vi "Math Rolling Buffer (by ref).vi"(0 "New Data In":sgl[][](array[numeric]), 1 "# Pts Read":u32, 3 "Number of Channels":i32=1, 4 "Sample Rate":dbl=2000.0, 5 "error in (no error)":errorcluster, 7 "Config.Test Limits":T1[](array[typedef]), 9 "Coefficients":cluster{"Coefficients":dbl[]}[](array[cluster]), 10 "Mode (Read)":T2=enum."Read") -> (14 "Buffer Out":sgl[][](array[numeric]), 15 "Data Indexes":i32[](array[numeric]), 16 "RMS":sgl[][](array[numeric]), 17 "PK-PK":sgl[][](array[numeric]), 18 "Frequency Data":sgl[][](array[numeric]), 19 "error out":errorcluster)   [LabVIEW 2019]
uses:
  Type Defs and Controls/Functional Global Control.ctl
  Type Defs and Controls/Test Limits.ctl
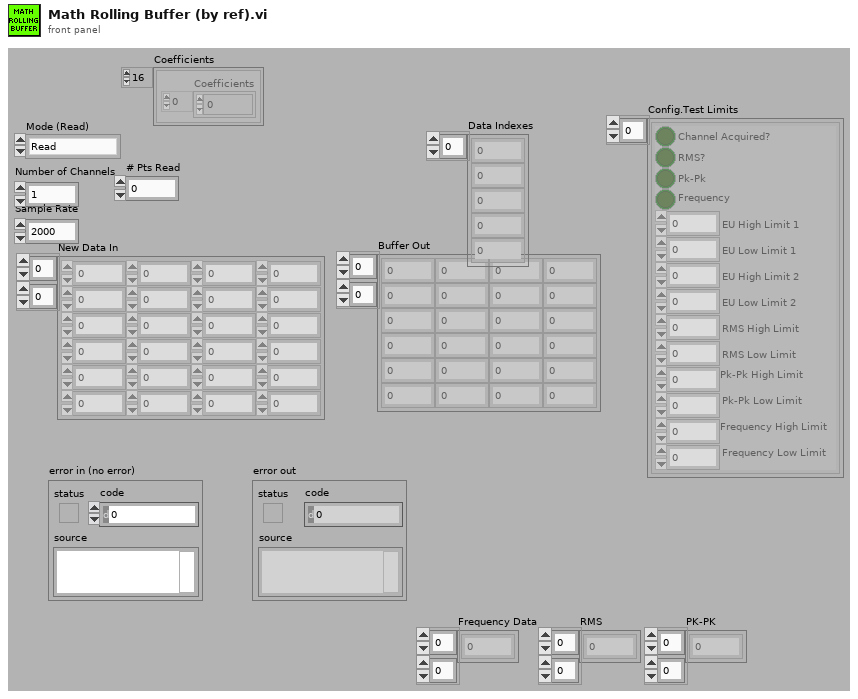
[diagram p1: front panel]
types:
  T1 = typedef "Test Limits.ctl" = cluster{"Channel Acquired?":bool, "RMS?":bool, "Pk-Pk":bool, "Frequency":bool, "EU High Limit 1":dbl, "EU Low Limit 1":dbl, "EU High Limit 2":dbl, "EU Low Limit 2":dbl, "RMS High Limit":dbl, "RMS Low Limit":dbl, "Pk-Pk High Limit ":dbl, "Pk-Pk Low Limit":dbl, "Frequency High Limit":dbl, "Frequency Low Limit":dbl}
  T2 = typedef "Functional Global Control.ctl" = enum16{"Nothing", "Init", "Read", "Write"}
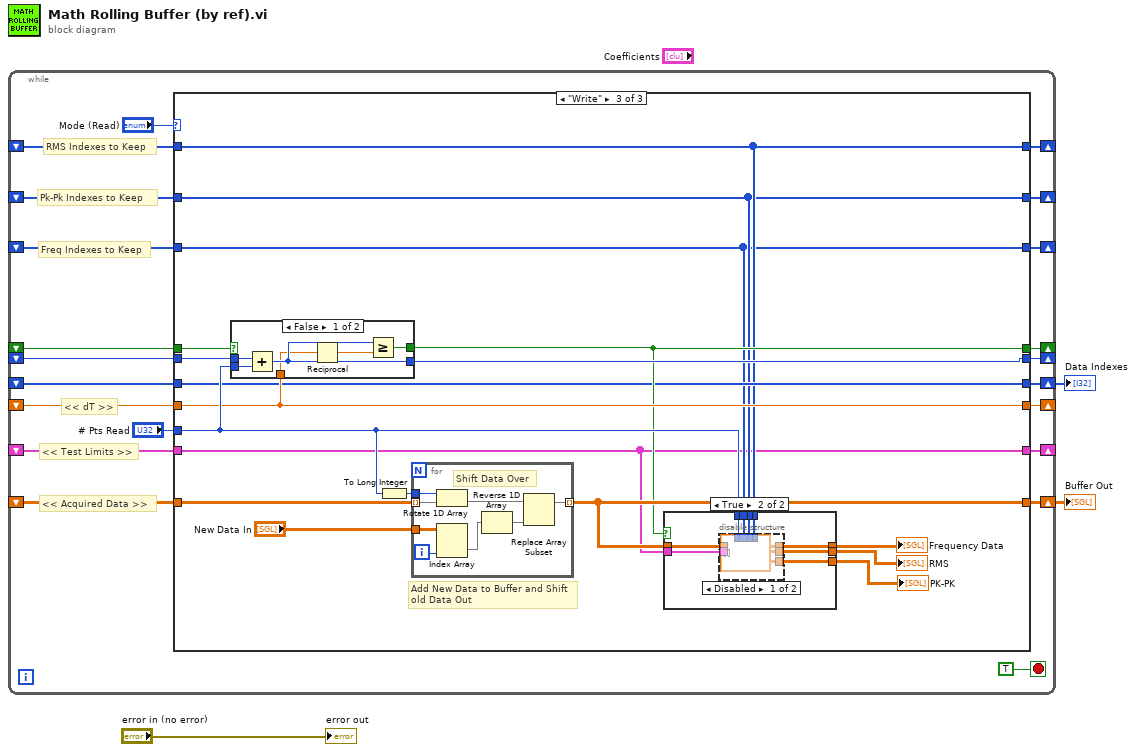
[diagram p0: block diagram]
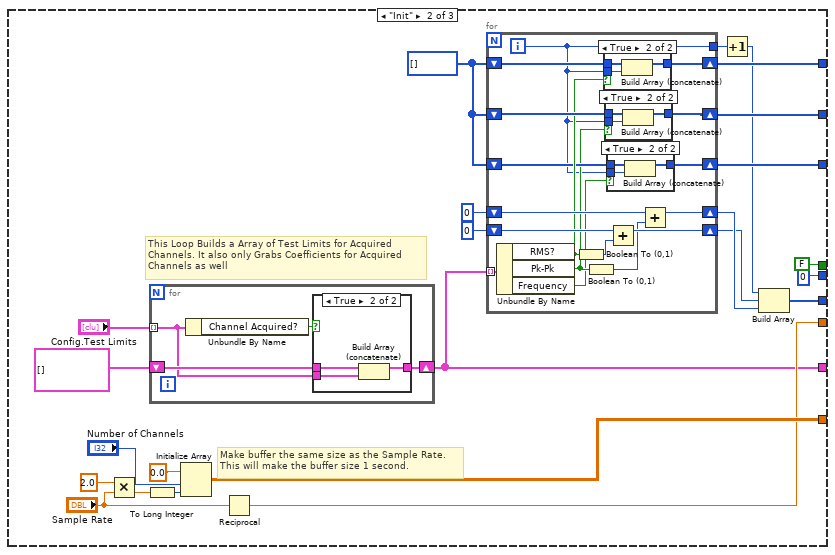
[diagram p3: hidden frame]
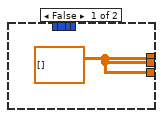
[diagram p8: hidden frame]
diagram:
  n1 = while {
    shift-right: [w22] -> w3
    shift-left: _ -> [w21]
    shift-right: [w20] -> _
    shift-left: _ -> [w19]
    shift-right: [w17] -> _
    shift-left: _ -> [w18]
    shift-right: [w14] -> _
    shift-left: _ -> [w15]
    shift-right: [w13] -> _
    shift-left: _ -> [w12]
    shift-right: [w11] -> w1
    shift-left: _ -> [w10]
    shift-right: [w9] -> _
    shift-left: _ -> [w6]
    shift-right: [w8] -> _
    shift-left: _ -> [w5]
    shift-right: [w7] -> _
    shift-left: _ -> [w4]
    stop <- TRUE stop-if-true
    # "Freq Indexes to Keep"
    # "Pk-Pk Indexes to Keep"
    # "RMS Indexes to Keep"
    # "<< dT >>"
    # "<< Test Limits >>"
    # "<< Acquired Data >>"
    n2 = case shown="\"Write\"" "Mode (Read)" {
      tunnel: [w33 w56 w110] -> w22
      tunnel: w21 -> [w33 _ w112]
      tunnel: [w32 w47 w95] -> w20
      tunnel: w19 -> [w32 _ w95]
      tunnel: w18 -> [w31 _ w105]
      tunnel: [w31 w52 w105] -> w17
      tunnel: "# Pts Read" -> [_ _ w108]
      tunnel: w15 -> [w30 _ w107]
      tunnel: [w30 FALSE w104] -> w14
      tunnel: [w29 0 w106] -> w13
      tunnel: w12 -> [w29 _ w109]
      tunnel: [w28 w45 w102] -> w11
      tunnel: w10 -> [w28 _ w102]
      tunnel: [w27 w40 w98] -> w9
      tunnel: [w26 w39 w97] -> w8
      tunnel: [w25 w38 w96] -> w7
      tunnel: w6 -> [w27 _ w98]
      tunnel: w5 -> [w26 _ w97]
      tunnel: w4 -> [w25 _ w96]
      frame Default {
      }
      frame "Init" {
        w41 = i32[] []
        # "This Loop Builds a Array of Test Limits for Acquired Channels. It also only Grabs Coefficients for Acquired Channels as well"
        # "Make buffer the same size as the Sample Rate.\nThis will make the buffer size 1 second."
        n3 = Multiply(x=2.0, y="Sample Rate") -> (x*y=w35:dbl)
        n4 = To Long Integer(number=w35) -> (32bit integer=w48:i32)
        n5 = for {
          tunnel: "Config.Test Limits" -> [w87] mode=indexing
          shift-right: [w89] -> w47
          shift-left: T1[] [] ("Config.Test Limits") -> [w90]
          n6 = Unbundle By Name(w87) -> ("Channel Acquired?"=w88:bool)
          n7 = case shown="True" w88 {
            tunnel: w90 -> [w91 w94]
            tunnel: [w91 w93] -> w89
            tunnel: w87 -> [_ w92]
            frame False {
            }
            frame True {
              n8 = Build Array (concatenate)(w94, w92) -> (w93:T1[])
            }
          }
        }
        n9 = Initialize Array(sgl 0.0, "Number of Channels", w48) -> (w56:sgl[][])
        n10 = Reciprocal(x="Sample Rate") -> (1/x=w52:dbl)
        n11 = for {
          tunnel: w47 -> [w74] mode=indexing
          shift-right: [w71] -> w42
          shift-left: 0 -> [w72]
          shift-right: [w69] -> w43
          shift-left: 0 -> [w70]
          shift-right: [w66] -> w40
          shift-left: w41 -> [w67]
          shift-right: [w61] -> w38
          shift-left: w41 -> [w62]
          shift-right: [w64] -> w39
          shift-left: w41 -> [w65]
          tunnel: [w58] -> w37
          i -> [w58]
          n12 = Unbundle By Name(w74) -> ("RMS?"=w63:bool, "Pk-Pk"=w60:bool, "Frequency"=w59:bool)
          n13 = Boolean To (0,1)(Boolean=w63) -> (0, 1=w73:i16)
          n14 = Boolean To (0,1)(Boolean=w60) -> (0, 1=w68:i16)
          n15 = case shown="True" w63 {
            tunnel: w67 -> [w83 w86]
            tunnel: [w83 w85] -> w66
            tunnel: w58 -> [_ w84]
            frame False {
            }
            frame True {
              n16 = Build Array (concatenate)(w86, w84) -> (w85:i32[])
            }
          }
          n17 = case shown="True" w60 {
            tunnel: w65 -> [w79 w82]
            tunnel: [w79 w81] -> w64
            tunnel: w58 -> [_ w80]
            frame False {
            }
            frame True {
              n18 = Build Array (concatenate)(w82, w80) -> (w81:i32[])
            }
          }
          n19 = case shown="True" w59 {
            tunnel: w62 -> [w75 w78]
            tunnel: [w75 w77] -> w61
            tunnel: w58 -> [_ w76]
            frame False {
            }
            frame True {
              n20 = Build Array (concatenate)(w78, w76) -> (w77:i32[])
            }
          }
          n21 = Add(x=w72, y=w73) -> (x+y=w71:i32)
          n22 = Add(x=w70, y=w68) -> (x+y=w69:i32)
        }
        n23 = Increment(x=w37) -> (x+1=w36:i32)
        n24 = Build Array(w36, w42, w43) -> (w45:i32[])
      }
      frame "Write" {
        # "Add New Data to Buffer and Shift old Data Out"
        n25 = case shown="False" w107 {
          selector: w107 -> [_ w131]
          tunnel: w109 -> [w129 w130]
          tunnel: w108 -> [w128 _]
          tunnel: [w127 w130] -> w106
          tunnel: w105 -> [w126 _]
          tunnel: [w124 w131] -> w104
          frame False {
            n26 = Add(x=w129, y=w128) -> (x+y=w127:u32)
            n27 = Reciprocal(x=w126) -> (1/x=w125:dbl)
            n28 = Greater Or Equal?(x=w127, y=w125) -> (x >= y?=w124:bool)
          }
          frame True {
          }
        }
        n29 = To Long Integer(number=w108) -> (32bit integer=w111:i32)
        n30 = for {
          tunnel: w112 -> [w139] mode=indexing
          tunnel: w111 -> [w138]
          tunnel: [w132] -> w110 mode=indexing
          tunnel: "New Data In" -> [w136]
          i -> [w135]
          # "Shift Data Over"
          n31 = Rotate 1D Array(1:w139, 2:w138) -> (0:w137:sgl[])
          n32 = Index Array(array=w136, index (col)=w135) -> (element=w134:sgl[])  [unwired: 1 in]
          n33 = Reverse 1D Array(array=w134) -> (reversed array=w133:sgl[])
          n34 = Replace Array Subset(array=w137, new element=w133) -> (w132:sgl[])  [unwired: 1 in]
        }
        n35 = case shown="True" w104 {
          tunnel: w110 -> [_ w122]
          tunnel: w108 -> [_ w121]
          tunnel: [w113 w120] -> w100
          tunnel: [w113 w119] -> w99
          tunnel: [w113 w118] -> w101
          tunnel: w98 -> [_ w117]
          tunnel: w97 -> [_ w116]
          tunnel: w96 -> [_ w115]
          tunnel: w95 -> [_ w114]
          frame False {
            w113 = sgl[][] [] ("Frequency Data")
          }
          frame True {
            n36 = disable-structure shown="Disabled" {
              disable-tunnel: w122 -> [_ _]
              disable-tunnel: w121 -> [_ _]
              disable-tunnel: [w123 _] -> w120
              disable-tunnel: [w123 _] -> w119
              disable-tunnel: [w123 _] -> w118
              disable-tunnel: w117 -> [_ _]
              disable-tunnel: w116 -> [_ _]
              disable-tunnel: w115 -> [_ _]
              disable-tunnel: w114 -> [_ _]
              frame Disabled {
                w123 = sgl[][] [] ("Frequency Data")
              }
              frame Enabled {
              }
            }
          }
        }
        "Frequency Data" <- w100
        "RMS" <- w99
        "PK-PK" <- w101
      }
    }
  }
  "Buffer Out" <- w3
  "Data Indexes" <- w1
  "error out" <- "error in (no error)"
